vi "Check_Z_settings.vi"(3 "PSOCT thickness":u32[](array[numeric]), 5 "Cut thickness":u32[](array[numeric]), 7 "2P thickness":u32[](array[numeric]), 8 "Error in":errorcluster, 9 "Pause?":bool[](array[boolean]), 10 "Cut_aft_2P?":bool[](array[boolean]), 11 "2P_cover_all?":bool[](array[boolean])) -> (0 "Error out":errorcluster, 1 "Exit?":bool)   [LabVIEW 2018]
uses:
  Controls/Queue Manager Actions.ctl
  Controls/MessagePacket.ctl
  Controls/FGV Actions.ctl
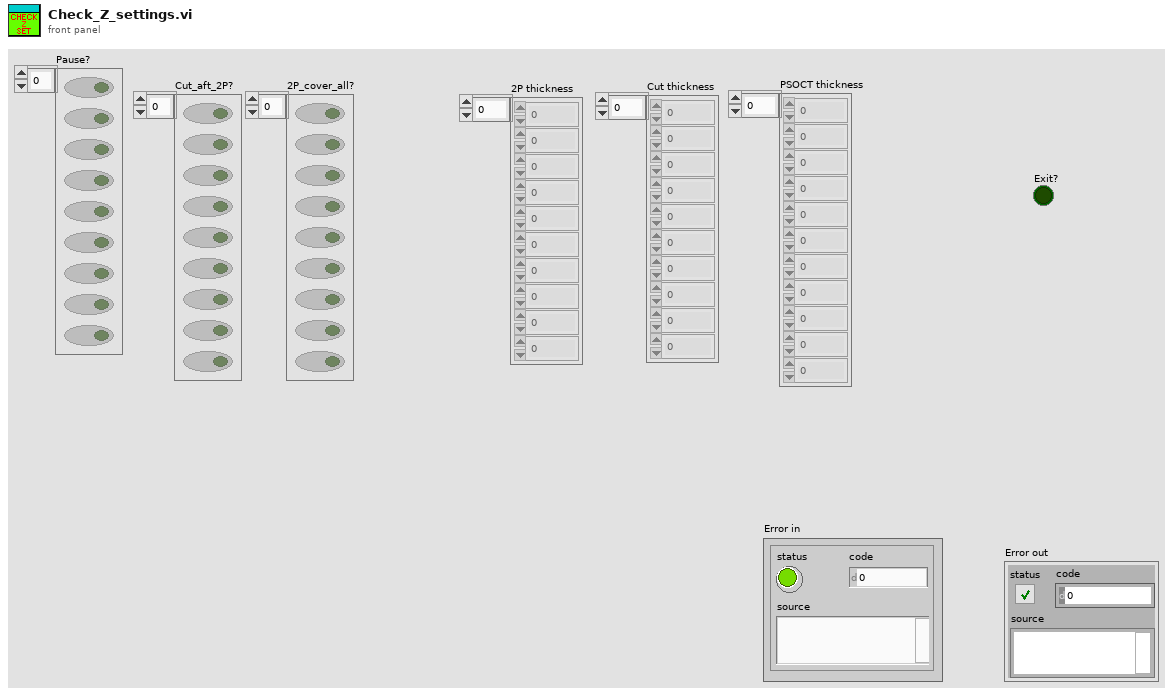
[diagram p1: front panel]
types:
  T1 = typedef "FGV Actions.ctl" = enum16{"Init", "Set", "Get", "Clear"}
  T2 = typedef "Queue Manager Actions.ctl" = enum16{"Init", "Enqueue", "Enqueue All", "Preview Queue", "Dequeue", "Get Status", "Flush Queue", "Flush All Queues", "Release All Queues", "Release Queue", "Enqueue at Opposite End"}
  T3 = typedef "MessagePacket.ctl" = cluster{"Message":string, "Parameter":variant}
  T4 = typedef "ScanType.ctl" = enum16{"Single Frame", "Continuous Frame", "ROI Line", "Vibratome", "Mosaic", "Mosaic + Slice"}
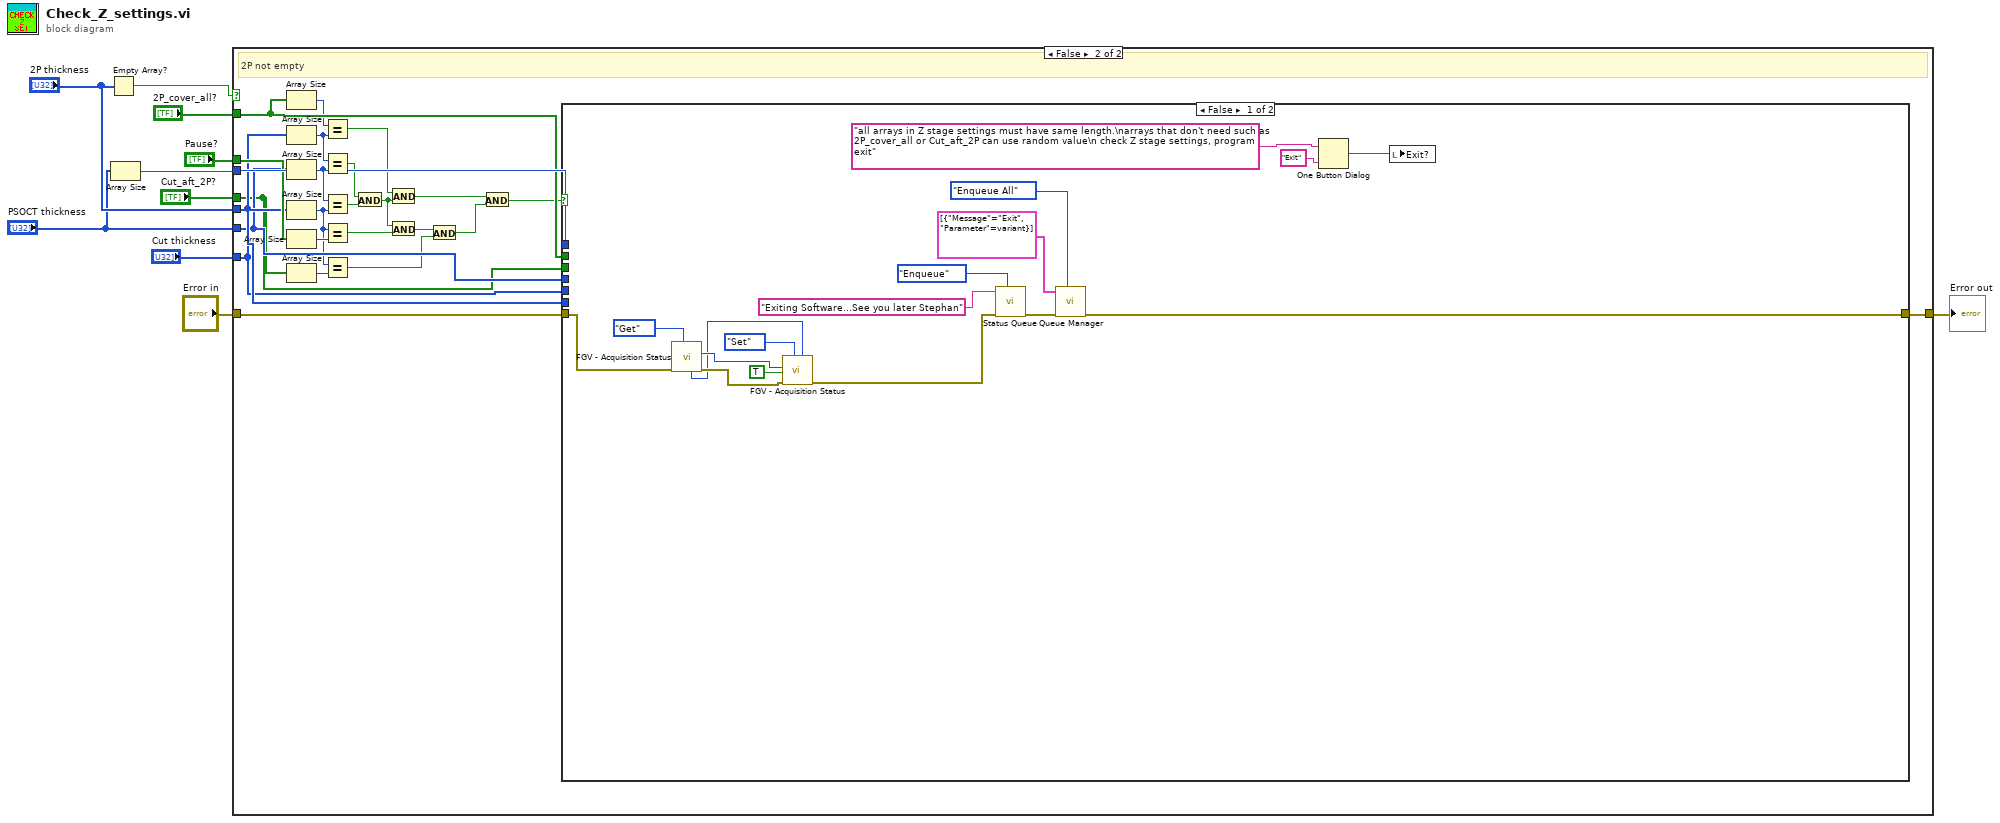
[diagram p0: block diagram]
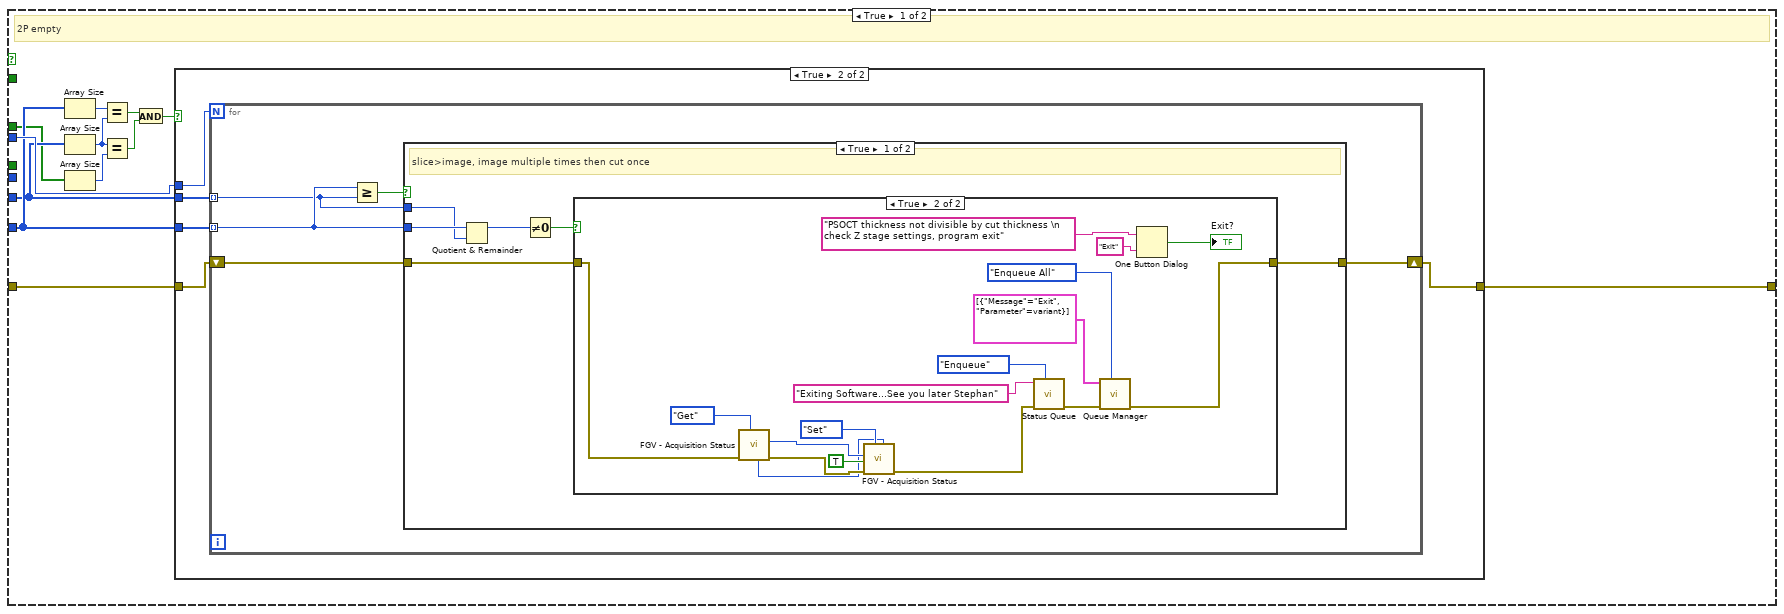
[diagram p2: hidden frame]
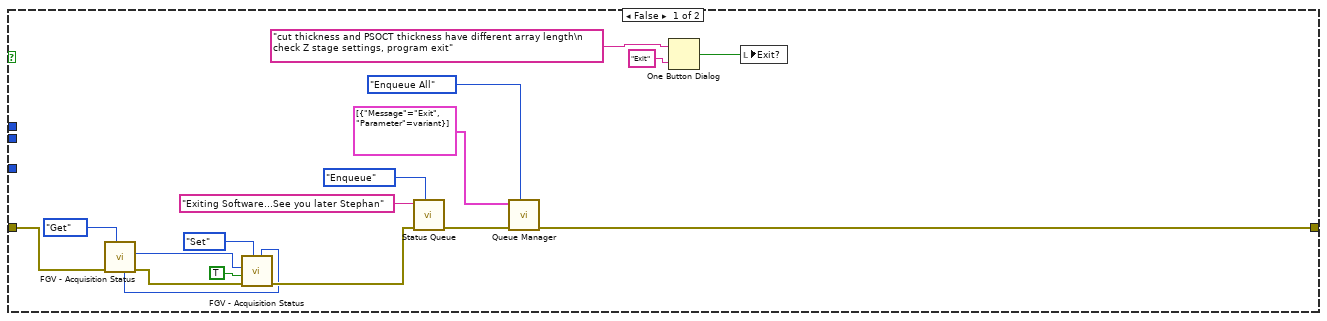
[diagram p3: hidden frame]
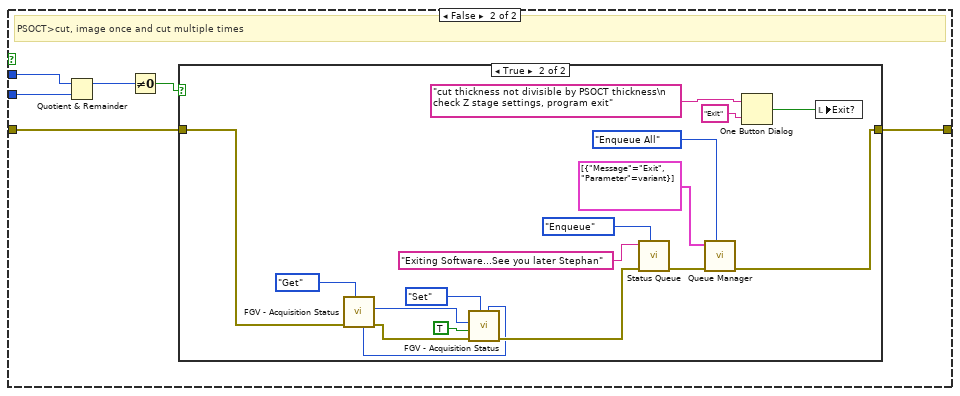
[diagram p5: hidden frame]
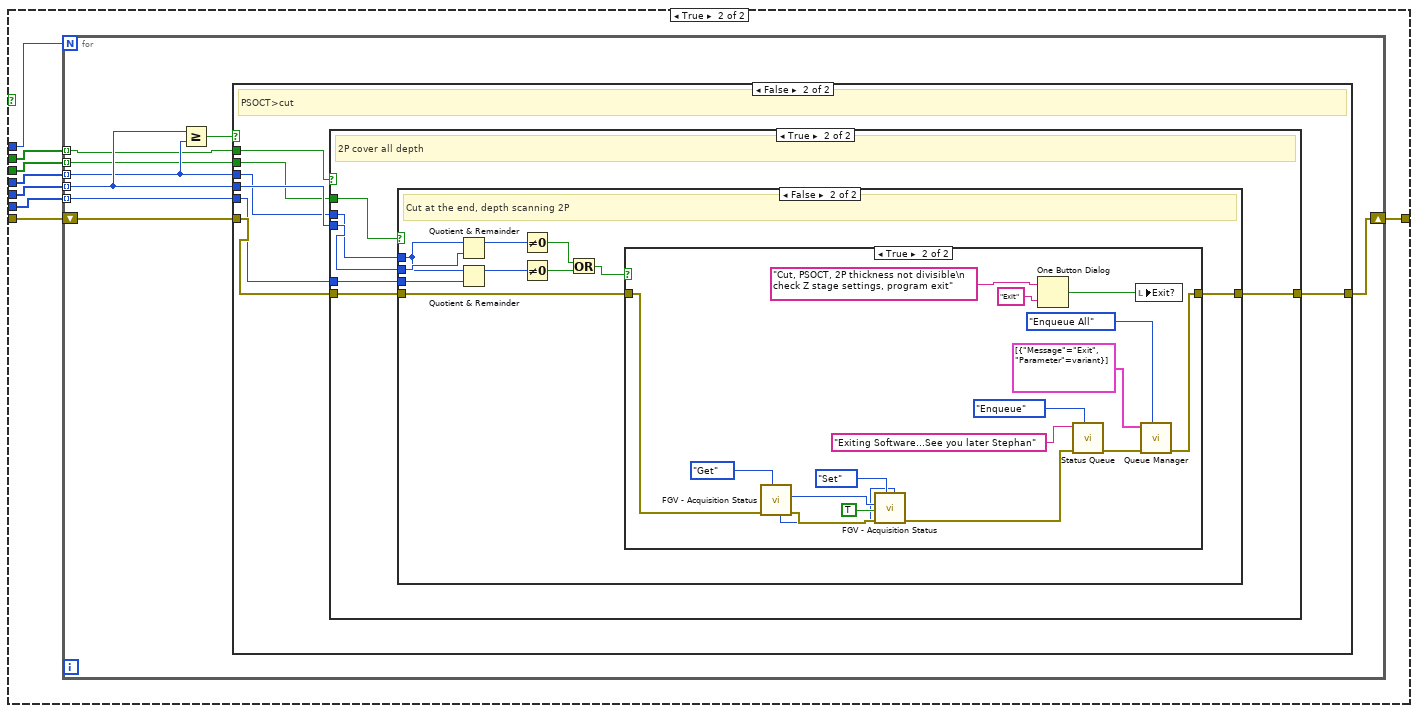
[diagram p7: hidden frame]
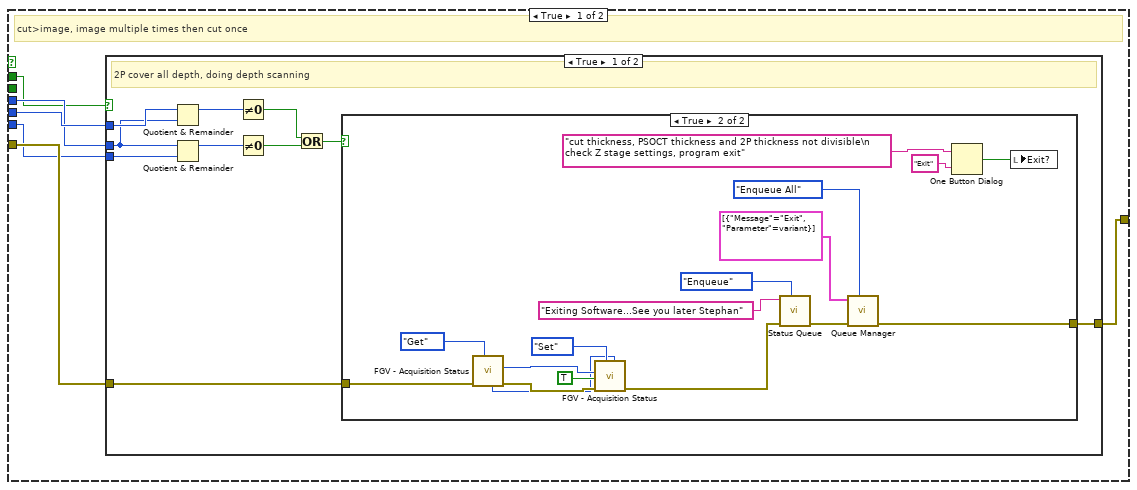
[diagram p8: hidden frame]
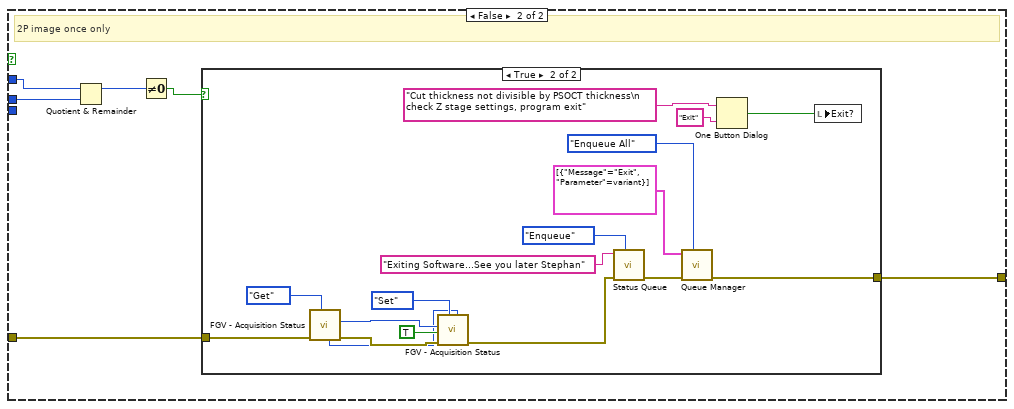
[diagram p10: hidden frame]
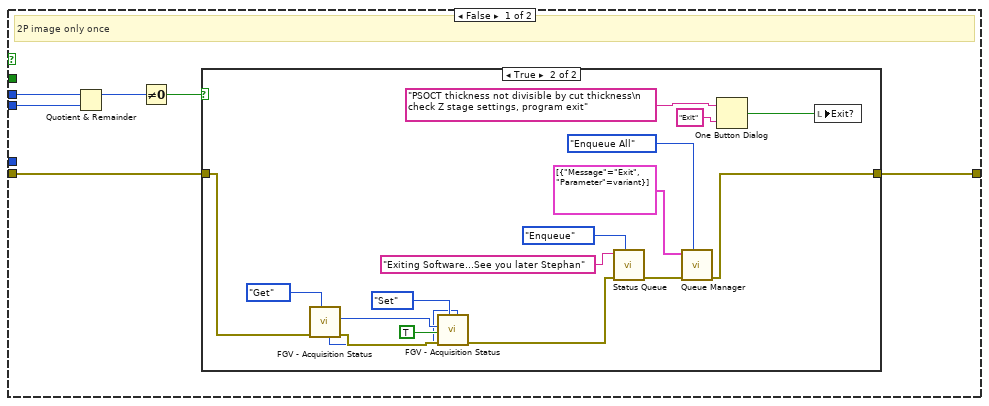
[diagram p12: hidden frame]
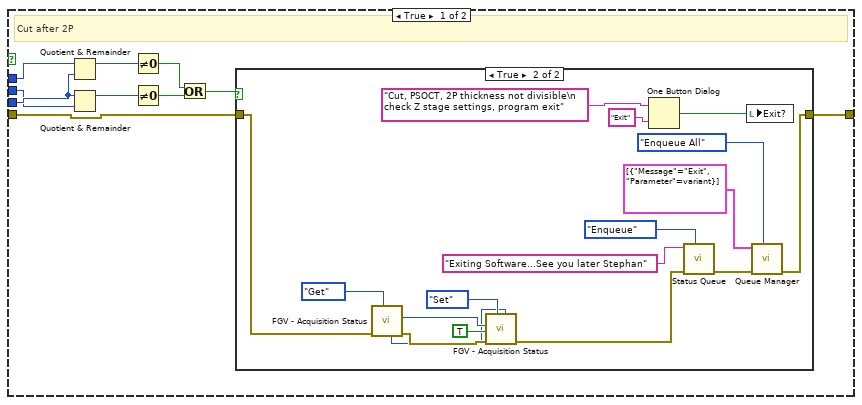
[diagram p14: hidden frame]
diagram:
  n1 = Empty Array?(array="2P thickness") -> (empty?=w2:bool)
  n2 = Array Size(array="PSOCT thickness") -> (size(s)=w8:i32)
  n3 = case shown="False" w2 {
    tunnel: "Cut thickness" -> [w19 w116]
    tunnel: "PSOCT thickness" -> [w18 w117]
    tunnel: w8 -> [w22 w122]
    tunnel: "Error in" -> [w21 w121]
    tunnel: [w20 w120] -> w9
    tunnel: "2P_cover_all?" -> [_ w109]
    tunnel: "2P thickness" -> [_ w118]
    tunnel: "Cut_aft_2P?" -> [_ w110]
    tunnel: "Pause?" -> [w16 w119]
    frame True {
      # "2P empty"
      n4 = Array Size(array=w19) -> (size(s)=w17:i32)
      n5 = Array Size(array=w18) -> (size(s)=w14:i32)
      n6 = Array Size(array=w16) -> (size(s)=w15:i32)
      n7 = Equal?(x=w17, y=w14) -> (x = y?=w12:bool)
      n8 = Equal?(x=w14, y=w15) -> (x = y?=w11:bool)
      n9 = And(x=w12, y=w11) -> (x .and. y?=w13:bool)
      n10 = case shown="True" w13 {
        tunnel: w19 -> [_ w44]
        tunnel: w18 -> [_ w43]
        tunnel: w22 -> [_ w42]
        tunnel: w21 -> [w39 w41]
        tunnel: [w24 w40] -> w20
        frame False {
          n11 = call "FGV - Acquisition Status.vi"("Actions"=FGV_Actions."Get", "Error In"=w39) -> ("Error Out"=w29:errorcluster, "Scan Type [Out]"=w27:T4, "mem loc out"=w25:i32)  [unwired: 6 in, 1 out]
          n12 = call "FGV - Acquisition Status.vi"("mem loc"=w25, "Actions"=FGV_Actions."Set", "Error In"=w29, "Quit status"=TRUE, "Scan Type [In]"=w27) -> ("Error Out"=w28:errorcluster)  [unwired: 3 in, 3 out]
          n13 = call "Status Queue.vi"("Action"=Queue_Manager_Actions."Enqueue", "Error In"=w28, "Status Message [In]"="Exiting Software...See you later Stephan") -> ("Error Out"=w33:errorcluster)  [unwired: 7 in, 1 out]
          n14 = call "Queue Manager.vi"("Action"=Queue_Manager_Actions."Enqueue All", "Error In"=w33, "Message Packet Array"=T3[] [{"Message"="Exit", "Parameter"=variant}] ("Message Packet [In]")) -> ("Error Out"=w24:errorcluster)  [unwired: 4 in, 4 out]
          n15 = One Button Dialog(message="cut thickness and PSOCT thickness have different array length\n check Z stage settings, program exit", button name ("OK")="Exit") -> (true=w23:bool)
          n16 = local write "Exit?"(w23) -> ()
        }
        frame True {
          n17 = for {
            N: w42 -> [_]
            tunnel: w44 -> [w49] mode=indexing
            tunnel: w43 -> [w48] mode=indexing
            shift-right: [w46] -> w40
            shift-left: w41 -> [w47]
            n18 = Greater Or Equal?(x=w49, y=w48) -> (x >= y?=w45:bool)
            n19 = case shown="True" w45 {
              tunnel: w49 -> [w55 w78]
              tunnel: w48 -> [w54 w79]
              tunnel: w47 -> [w51 w75]
              tunnel: [w50 w74] -> w46
              frame True {
                # "slice>image, image multiple times then cut once"
                n20 = Quotient & Remainder(x=w55, y=w54) -> (x-y*floor(x/y)=w53:u32)  [unwired: 1 out]
                n21 = Not Equal To 0?(x=w53) -> (x != 0?=w52:bool)
                n22 = case shown="True" w52 {
                  tunnel: w51 -> [w56 w58]
                  tunnel: [w56 w57] -> w50
                  frame False {
                  }
                  frame True {
                    n23 = call "FGV - Acquisition Status.vi"("Actions"=FGV_Actions."Get", "Error In"=w58) -> ("Error Out"=w63:errorcluster, "Scan Type [Out]"=w61:T4, "mem loc out"=w59:i32)  [unwired: 6 in, 1 out]
                    n24 = call "FGV - Acquisition Status.vi"("mem loc"=w59, "Actions"=FGV_Actions."Set", "Error In"=w63, "Quit status"=TRUE, "Scan Type [In]"=w61) -> ("Error Out"=w62:errorcluster)  [unwired: 3 in, 3 out]
                    n25 = call "Status Queue.vi"("Action"=Queue_Manager_Actions."Enqueue", "Error In"=w62, "Status Message [In]"="Exiting Software...See you later Stephan") -> ("Error Out"=w67:errorcluster)  [unwired: 7 in, 1 out]
                    n26 = call "Queue Manager.vi"("Action"=Queue_Manager_Actions."Enqueue All", "Error In"=w67, "Message Packet Array"=T3[] [{"Message"="Exit", "Parameter"=variant}] ("Message Packet [In]")) -> ("Error Out"=w57:errorcluster)  [unwired: 4 in, 4 out]
                    n27 = One Button Dialog(message="PSOCT thickness not divisible by cut thickness \n check Z stage settings, program exit", button name ("OK")="Exit") -> (true=→"Exit?":bool)
                  }
                }
              }
              frame False {
                # "PSOCT>cut, image once and cut multiple times"
                n28 = Quotient & Remainder(x=w79, y=w78) -> (x-y*floor(x/y)=w77:u32)  [unwired: 1 out]
                n29 = Not Equal To 0?(x=w77) -> (x != 0?=w76:bool)
                n30 = case shown="True" w76 {
                  tunnel: w75 -> [w80 w83]
                  tunnel: [w80 w82] -> w74
                  frame False {
                  }
                  frame True {
                    n31 = call "FGV - Acquisition Status.vi"("Actions"=FGV_Actions."Get", "Error In"=w83) -> ("Error Out"=w88:errorcluster, "Scan Type [Out]"=w86:T4, "mem loc out"=w84:i32)  [unwired: 6 in, 1 out]
                    n32 = call "FGV - Acquisition Status.vi"("mem loc"=w84, "Actions"=FGV_Actions."Set", "Error In"=w88, "Quit status"=TRUE, "Scan Type [In]"=w86) -> ("Error Out"=w87:errorcluster)  [unwired: 3 in, 3 out]
                    n33 = call "Status Queue.vi"("Action"=Queue_Manager_Actions."Enqueue", "Error In"=w87, "Status Message [In]"="Exiting Software...See you later Stephan") -> ("Error Out"=w92:errorcluster)  [unwired: 7 in, 1 out]
                    n34 = call "Queue Manager.vi"("Action"=Queue_Manager_Actions."Enqueue All", "Error In"=w92, "Message Packet Array"=T3[] [{"Message"="Exit", "Parameter"=variant}] ("Message Packet [In]")) -> ("Error Out"=w82:errorcluster)  [unwired: 4 in, 4 out]
                    n35 = One Button Dialog(message="cut thickness not divisible by PSOCT thickness\n check Z stage settings, program exit", button name ("OK")="Exit") -> (true=w81:bool)
                    n36 = local write "Exit?"(w81) -> ()
                  }
                }
              }
            }
          }
        }
      }
    }
    frame False {
      # "2P not empty"
      n37 = Array Size(array=w109) -> (size(s)=w105:i32)
      n38 = Array Size(array=w116) -> (size(s)=w106:i32)
      n39 = Array Size(array=w117) -> (size(s)=w114:i32)
      n40 = Array Size(array=w118) -> (size(s)=w107:i32)
      n41 = Array Size(array=w119) -> (size(s)=w115:i32)
      n42 = Array Size(array=w110) -> (size(s)=w108:i32)
      n43 = Equal?(x=w105, y=w106) -> (x = y?=w104:bool)
      n44 = Equal?(x=w106, y=w114) -> (x = y?=w113:bool)
      n45 = Equal?(x=w114, y=w107) -> (x = y?=w112:bool)
      n46 = Equal?(x=w107, y=w115) -> (x = y?=w111:bool)
      n47 = Equal?(x=w107, y=w108) -> (x = y?=w102:bool)
      n48 = And(x=w113, y=w112) -> (x .and. y?=w103:bool)
      n49 = And(x=w104, y=w103) -> (x .and. y?=w99:bool)
      n50 = And(x=w103, y=w111) -> (x .and. y?=w101:bool)
      n51 = And(x=w101, y=w102) -> (x .and. y?=w100:bool)
      n52 = And(x=w99, y=w100) -> (x .and. y?=w98:bool)
      n53 = case shown="False" w98 {
        tunnel: w122 -> [_ w147]
        tunnel: w121 -> [w139 w146]
        tunnel: [w138 w145] -> w120
        tunnel: w109 -> [_ w144]
        tunnel: w110 -> [_ w143]
        tunnel: w118 -> [_ w142]
        tunnel: w117 -> [_ w141]
        tunnel: w116 -> [_ w140]
        frame False {
          n54 = call "FGV - Acquisition Status.vi"("Actions"=FGV_Actions."Get", "Error In"=w139) -> ("Error Out"=w128:errorcluster, "Scan Type [Out]"=w126:T4, "mem loc out"=w124:i32)  [unwired: 6 in, 1 out]
          n55 = call "FGV - Acquisition Status.vi"("mem loc"=w124, "Actions"=FGV_Actions."Set", "Error In"=w128, "Quit status"=TRUE, "Scan Type [In]"=w126) -> ("Error Out"=w127:errorcluster)  [unwired: 3 in, 3 out]
          n56 = call "Status Queue.vi"("Action"=Queue_Manager_Actions."Enqueue", "Error In"=w127, "Status Message [In]"="Exiting Software...See you later Stephan") -> ("Error Out"=w132:errorcluster)  [unwired: 7 in, 1 out]
          n57 = call "Queue Manager.vi"("Action"=Queue_Manager_Actions."Enqueue All", "Error In"=w132, "Message Packet Array"=T3[] [{"Message"="Exit", "Parameter"=variant}] ("Message Packet [In]")) -> ("Error Out"=w138:errorcluster)  [unwired: 4 in, 4 out]
          n58 = One Button Dialog(message="all arrays in Z stage settings must have same length.\narrays that don't need such as 2P_cover_all or Cut_aft_2P can use random value\n check Z stage settings, program exit", button name ("OK")="Exit") -> (true=w123:bool)
          n59 = local write "Exit?"(w123) -> ()
        }
        frame True {
          n60 = for {
            N: w147 -> [_]
            tunnel: w140 -> [w155] mode=indexing
            tunnel: w141 -> [w154] mode=indexing
            shift-right: [w152] -> w145
            shift-left: w146 -> [w153]
            tunnel: w144 -> [w151] mode=indexing
            tunnel: w142 -> [w149] mode=indexing
            tunnel: w143 -> [w150] mode=indexing
            n61 = Greater Or Equal?(x=w155, y=w154) -> (x >= y?=w148:bool)
            n62 = case shown="False" w148 {
              tunnel: w155 -> [w159 w218]
              tunnel: w154 -> [w158 w217]
              tunnel: w153 -> [w161 w220]
              tunnel: [w160 w219] -> w152
              tunnel: w151 -> [w157 w216]
              tunnel: w150 -> [_ w215]
              tunnel: w149 -> [w156 w214]
              frame True {
                # "cut>image, image multiple times then cut once"
                n63 = case shown="True" w157 {
                  tunnel: w161 -> [w163 w191]
                  tunnel: [w162 w190] -> w160
                  tunnel: w159 -> [w171 w195]
                  tunnel: w158 -> [w170 w194]
                  tunnel: w156 -> [w169 _]
                  frame True {
                    # "2P cover all depth, doing depth scanning"
                    n64 = Quotient & Remainder(x=w171, y=w170) -> (x-y*floor(x/y)=w167:u32)  [unwired: 1 out]
                    n65 = Quotient & Remainder(x=w170, y=w169) -> (x-y*floor(x/y)=w168:u32)  [unwired: 1 out]
                    n66 = Not Equal To 0?(x=w167) -> (x != 0?=w165:bool)
                    n67 = Not Equal To 0?(x=w168) -> (x != 0?=w164:bool)
                    n68 = Or(x=w165, y=w164) -> (x .or. y?=w166:bool)
                    n69 = case shown="True" w166 {
                      tunnel: w163 -> [w172 w175]
                      tunnel: [w172 w174] -> w162
                      frame False {
                      }
                      frame True {
                        n70 = call "FGV - Acquisition Status.vi"("Actions"=FGV_Actions."Get", "Error In"=w175) -> ("Error Out"=w180:errorcluster, "Scan Type [Out]"=w178:T4, "mem loc out"=w176:i32)  [unwired: 6 in, 1 out]
                        n71 = call "FGV - Acquisition Status.vi"("mem loc"=w176, "Actions"=FGV_Actions."Set", "Error In"=w180, "Quit status"=TRUE, "Scan Type [In]"=w178) -> ("Error Out"=w179:errorcluster)  [unwired: 3 in, 3 out]
                        n72 = call "Status Queue.vi"("Action"=Queue_Manager_Actions."Enqueue", "Error In"=w179, "Status Message [In]"="Exiting Software...See you later Stephan") -> ("Error Out"=w184:errorcluster)  [unwired: 7 in, 1 out]
                        n73 = call "Queue Manager.vi"("Action"=Queue_Manager_Actions."Enqueue All", "Error In"=w184, "Message Packet Array"=T3[] [{"Message"="Exit", "Parameter"=variant}] ("Message Packet [In]")) -> ("Error Out"=w174:errorcluster)  [unwired: 4 in, 4 out]
                        n74 = One Button Dialog(message="cut thickness, PSOCT thickness and 2P thickness not divisible\n check Z stage settings, program exit", button name ("OK")="Exit") -> (true=w173:bool)
                        n75 = local write "Exit?"(w173) -> ()
                      }
                    }
                  }
                  frame False {
                    # "2P image once only"
                    n76 = Quotient & Remainder(x=w195, y=w194) -> (x-y*floor(x/y)=w193:u32)  [unwired: 1 out]
                    n77 = Not Equal To 0?(x=w193) -> (x != 0?=w192:bool)
                    n78 = case shown="True" w192 {
                      tunnel: [w196 w199] -> w190
                      tunnel: w191 -> [w196 w198]
                      frame False {
                      }
                      frame True {
                        n79 = call "FGV - Acquisition Status.vi"("Actions"=FGV_Actions."Get", "Error In"=w198) -> ("Error Out"=w204:errorcluster, "Scan Type [Out]"=w202:T4, "mem loc out"=w200:i32)  [unwired: 6 in, 1 out]
                        n80 = call "FGV - Acquisition Status.vi"("mem loc"=w200, "Actions"=FGV_Actions."Set", "Error In"=w204, "Quit status"=TRUE, "Scan Type [In]"=w202) -> ("Error Out"=w203:errorcluster)  [unwired: 3 in, 3 out]
                        n81 = call "Status Queue.vi"("Action"=Queue_Manager_Actions."Enqueue", "Error In"=w203, "Status Message [In]"="Exiting Software...See you later Stephan") -> ("Error Out"=w208:errorcluster)  [unwired: 7 in, 1 out]
                        n82 = call "Queue Manager.vi"("Action"=Queue_Manager_Actions."Enqueue All", "Error In"=w208, "Message Packet Array"=T3[] [{"Message"="Exit", "Parameter"=variant}] ("Message Packet [In]")) -> ("Error Out"=w199:errorcluster)  [unwired: 4 in, 4 out]
                        n83 = One Button Dialog(message="Cut thickness not divisible by PSOCT thickness\n check Z stage settings, program exit", button name ("OK")="Exit") -> (true=w197:bool)
                        n84 = local write "Exit?"(w197) -> ()
                      }
                    }
                  }
                }
              }
              frame False {
                # "PSOCT>cut"
                n85 = case shown="True" w216 {
                  tunnel: w220 -> [w225 w250]
                  tunnel: [w224 w249] -> w219
                  tunnel: w218 -> [w221 w248]
                  tunnel: w217 -> [w222 w246]
                  tunnel: w215 -> [_ w247]
                  tunnel: w214 -> [_ w245]
                  frame False {
                    # "2P image only once"
                    n86 = Quotient & Remainder(x=w222, y=w221) -> (x-y*floor(x/y)=w226:u32)  [unwired: 1 out]
                    n87 = Not Equal To 0?(x=w226) -> (x != 0?=w223:bool)
                    n88 = case shown="True" w223 {
                      tunnel: w225 -> [w227 w230]
                      tunnel: [w227 w229] -> w224
                      frame False {
                      }
                      frame True {
                        n89 = call "FGV - Acquisition Status.vi"("Actions"=FGV_Actions."Get", "Error In"=w230) -> ("Error Out"=w235:errorcluster, "Scan Type [Out]"=w233:T4, "mem loc out"=w231:i32)  [unwired: 6 in, 1 out]
                        n90 = call "FGV - Acquisition Status.vi"("mem loc"=w231, "Actions"=FGV_Actions."Set", "Error In"=w235, "Quit status"=TRUE, "Scan Type [In]"=w233) -> ("Error Out"=w234:errorcluster)  [unwired: 3 in, 3 out]
                        n91 = call "Status Queue.vi"("Action"=Queue_Manager_Actions."Enqueue", "Error In"=w234, "Status Message [In]"="Exiting Software...See you later Stephan") -> ("Error Out"=w239:errorcluster)  [unwired: 7 in, 1 out]
                        n92 = call "Queue Manager.vi"("Action"=Queue_Manager_Actions."Enqueue All", "Error In"=w239, "Message Packet Array"=T3[] [{"Message"="Exit", "Parameter"=variant}] ("Message Packet [In]")) -> ("Error Out"=w229:errorcluster)  [unwired: 4 in, 4 out]
                        n93 = One Button Dialog(message="PSOCT thickness not divisible by cut thickness\n check Z stage settings, program exit", button name ("OK")="Exit") -> (true=w228:bool)
                        n94 = local write "Exit?"(w228) -> ()
                      }
                    }
                  }
                  frame True {
                    # "2P cover all depth"
                    n95 = case shown="False" w247 {
                      tunnel: w250 -> [w255 w283]
                      tunnel: [w254 w282] -> w249
                      tunnel: w248 -> [w251 w281]
                      tunnel: w246 -> [w253 w280]
                      tunnel: w245 -> [w252 w279]
                      frame True {
                        # "Cut after 2P"
                        n96 = Quotient & Remainder(x=w253, y=w252) -> (x-y*floor(x/y)=w259:u32)  [unwired: 1 out]
                        n97 = Quotient & Remainder(x=w252, y=w251) -> (x-y*floor(x/y)=w260:u32)  [unwired: 1 out]
                        n98 = Not Equal To 0?(x=w259) -> (x != 0?=w257:bool)
                        n99 = Not Equal To 0?(x=w260) -> (x != 0?=w256:bool)
                        n100 = Or(x=w257, y=w256) -> (x .or. y?=w258:bool)
                        n101 = case shown="True" w258 {
                          tunnel: w255 -> [w261 w264]
                          tunnel: [w261 w263] -> w254
                          frame False {
                          }
                          frame True {
                            n102 = call "FGV - Acquisition Status.vi"("Actions"=FGV_Actions."Get", "Error In"=w264) -> ("Error Out"=w269:errorcluster, "Scan Type [Out]"=w267:T4, "mem loc out"=w265:i32)  [unwired: 6 in, 1 out]
                            n103 = call "FGV - Acquisition Status.vi"("mem loc"=w265, "Actions"=FGV_Actions."Set", "Error In"=w269, "Quit status"=TRUE, "Scan Type [In]"=w267) -> ("Error Out"=w268:errorcluster)  [unwired: 3 in, 3 out]
                            n104 = One Button Dialog(message="Cut, PSOCT, 2P thickness not divisible\n check Z stage settings, program exit", button name ("OK")="Exit") -> (true=w262:bool)
                            n105 = call "Status Queue.vi"("Action"=Queue_Manager_Actions."Enqueue", "Error In"=w268, "Status Message [In]"="Exiting Software...See you later Stephan") -> ("Error Out"=w273:errorcluster)  [unwired: 7 in, 1 out]
                            n106 = local write "Exit?"(w262) -> ()
                            n107 = call "Queue Manager.vi"("Action"=Queue_Manager_Actions."Enqueue All", "Error In"=w273, "Message Packet Array"=T3[] [{"Message"="Exit", "Parameter"=variant}] ("Message Packet [In]")) -> ("Error Out"=w263:errorcluster)  [unwired: 4 in, 4 out]
                          }
                        }
                      }
                      frame False {
                        # "Cut at the end, depth scanning 2P"
                        n108 = Quotient & Remainder(x=w280, y=w281) -> (x-y*floor(x/y)=w287:u32)  [unwired: 1 out]
                        n109 = Quotient & Remainder(x=w280, y=w279) -> (x-y*floor(x/y)=w288:u32)  [unwired: 1 out]
                        n110 = Not Equal To 0?(x=w287) -> (x != 0?=w285:bool)
                        n111 = Not Equal To 0?(x=w288) -> (x != 0?=w284:bool)
                        n112 = Or(x=w285, y=w284) -> (x .or. y?=w286:bool)
                        n113 = case shown="True" w286 {
                          tunnel: w283 -> [w289 w292]
                          tunnel: [w289 w291] -> w282
                          frame False {
                          }
                          frame True {
                            n114 = call "FGV - Acquisition Status.vi"("Actions"=FGV_Actions."Get", "Error In"=w292) -> ("Error Out"=w297:errorcluster, "Scan Type [Out]"=w295:T4, "mem loc out"=w293:i32)  [unwired: 6 in, 1 out]
                            n115 = call "FGV - Acquisition Status.vi"("mem loc"=w293, "Actions"=FGV_Actions."Set", "Error In"=w297, "Quit status"=TRUE, "Scan Type [In]"=w295) -> ("Error Out"=w296:errorcluster)  [unwired: 3 in, 3 out]
                            n116 = One Button Dialog(message="Cut, PSOCT, 2P thickness not divisible\n check Z stage settings, program exit", button name ("OK")="Exit") -> (true=w290:bool)
                            n117 = call "Status Queue.vi"("Action"=Queue_Manager_Actions."Enqueue", "Error In"=w296, "Status Message [In]"="Exiting Software...See you later Stephan") -> ("Error Out"=w301:errorcluster)  [unwired: 7 in, 1 out]
                            n118 = local write "Exit?"(w290) -> ()
                            n119 = call "Queue Manager.vi"("Action"=Queue_Manager_Actions."Enqueue All", "Error In"=w301, "Message Packet Array"=T3[] [{"Message"="Exit", "Parameter"=variant}] ("Message Packet [In]")) -> ("Error Out"=w291:errorcluster)  [unwired: 4 in, 4 out]
                          }
                        }
                      }
                    }
                  }
                }
              }
            }
          }
        }
      }
    }
  }
  "Error out" <- w9
